vi "Write Append.vi"(8 "error in (no error)":errorcluster, 10 "Append (0=F)":i32, 11 "Data in":refnum<class "LV-Data.lvclass">) -> (0 "error out":errorcluster, 3 "Data out":refnum<class "LV-Data.lvclass">)   [LabVIEW 2019, in "LV-Data.lvclass"]
uses:
  LV-Data.lvclass
  LV-Data.lvclass/LV-Data.ctl
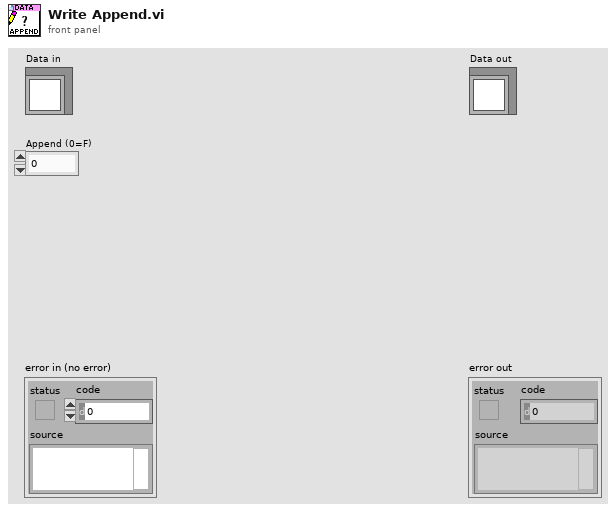
[diagram p1: front panel]
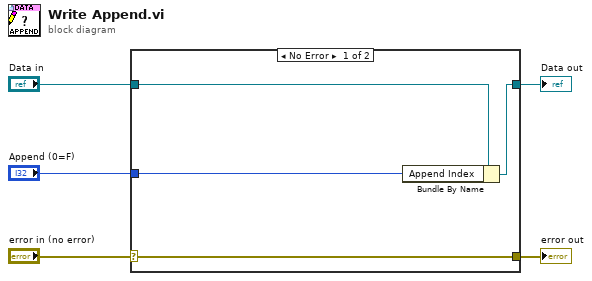
[diagram p0: block diagram]
diagram:
  n1 = case shown="No Error" "error in (no error)" {
    selector: "error in (no error)" -> [w9 w10]
    tunnel: [w9 w10] -> w4
    tunnel: [w7 w11] -> w2
    tunnel: "Data in" -> [w8 w11]
    tunnel: "Append (0=F)" -> [w6 _]
    frame No Error {
      n2 = Bundle By Name(cluster=w8, "Append Index"=w6) -> (w7:refnum<class "LV-Data.lvclass">)
    }
    frame Error {
    }
  }
  "error out" <- w4
  "Data out" <- w2
